vi "ReloaderMecanism.vi"() -> ()   [LabVIEW 2016]
uses:
  Globals/DIO.ctl
  Globals/Globals.vi
  Globals/InputValues.vi
panel:
  in  "wait":dbl
  out "Boolean":bool
  in  "Numeric":dbl
  out "Step even":bool
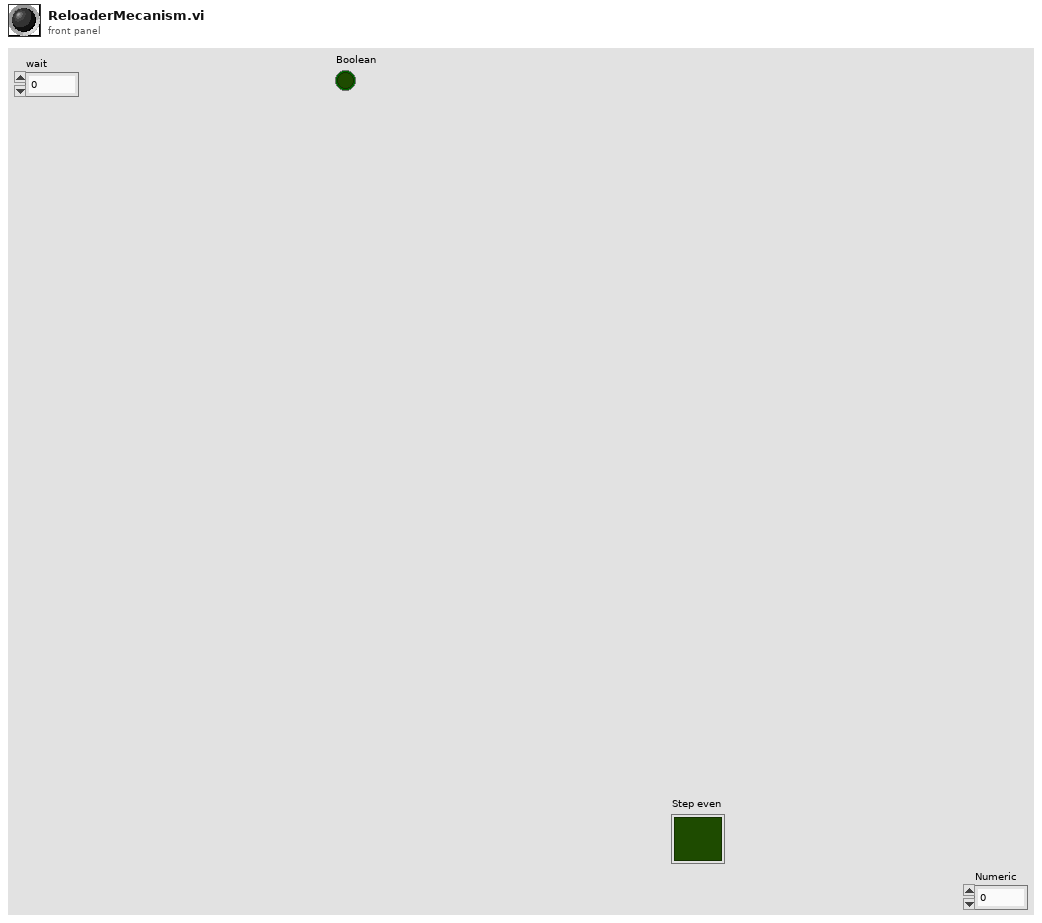
[diagram p1: front panel]
types:
  T1 = typedef "DIO.ctl" = string
  T2 = typedef "WPI_ServoDeviceRef.ctl" = cluster{"DeviceStatus":errorcluster, "PWM Channel":T3, "DeadBand":T4}
  T3 = typedef "FPGA_DIOPWMChannel.ctl" = enum8{"PWM 0", "PWM 1", "PWM 2", "PWM 3", "PWM 4", "PWM 5", "PWM 6", "PWM 7", "PWM 8", "PWM 9", "PWM MXP 0", "PWM MXP 1", "PWM MXP 2", "PWM MXP 3", "PWM MXP 4", "PWM MXP 5", "PWM MXP 6", "PWM MXP 7", "PWM MXP 8", "PWM MXP 9", "Invalid"}
  T4 = typedef "WPI_PWMDeadband.ctl" = cluster{"Name":string, "maxPositivePwm":i32, "minPositivePwm":i32, "centerPwm":i32, "maxNegativePwm":i32, "minNegativePwm":i32, "angularRange":u16}
  T5 = typedef "WPI_DigitalOutputDevRef.ctl" = cluster{"DIO Channel":T6, "DevStatus":errorcluster}
  T6 = typedef "FPGA_DIOChannel.ctl" = enum8{"DIO 0", "DIO 1", "DIO 2", "DIO 3", "DIO 4", "DIO 5", "DIO 6", "DIO 7", "DIO 8", "DIO 9", "DIO MXP 0", "DIO MXP 1", "DIO MXP 2", "DIO MXP 3", "DIO MXP 4", "DIO MXP 5", "DIO MXP 6", "DIO MXP 7", "DIO MXP 8", "DIO MXP 9", "DIO MXP 10", "DIO MXP 11", "DIO MXP 12", "DIO MXP 13", "DIO MXP 14", "DIO MXP 15", "SPI Port CS1", "SPI Port CS2", "SPI Port CS3", "SPI Port MISO", "SPI Port MOSI", "Invalid"}
  T7 = typedef "WPI_MotorControlDeviceRef.ctl" = cluster{"DeviceStatus":errorcluster, "Type":T8, "PWM":cluster{"PWM Channel":T3, "DeadBand":T4}, "CAN":cluster{"Device Number":u8, "SetOutput VI Ref":variant, "GetOutput VI Ref":variant, "Enable VI Ref":variant, "Disable VI Ref":variant, "Data":variant}, "Invert":bool}
  T8 = typedef "WPI_MotorControlType.ctl" = enum16{"PWM", "CAN"}
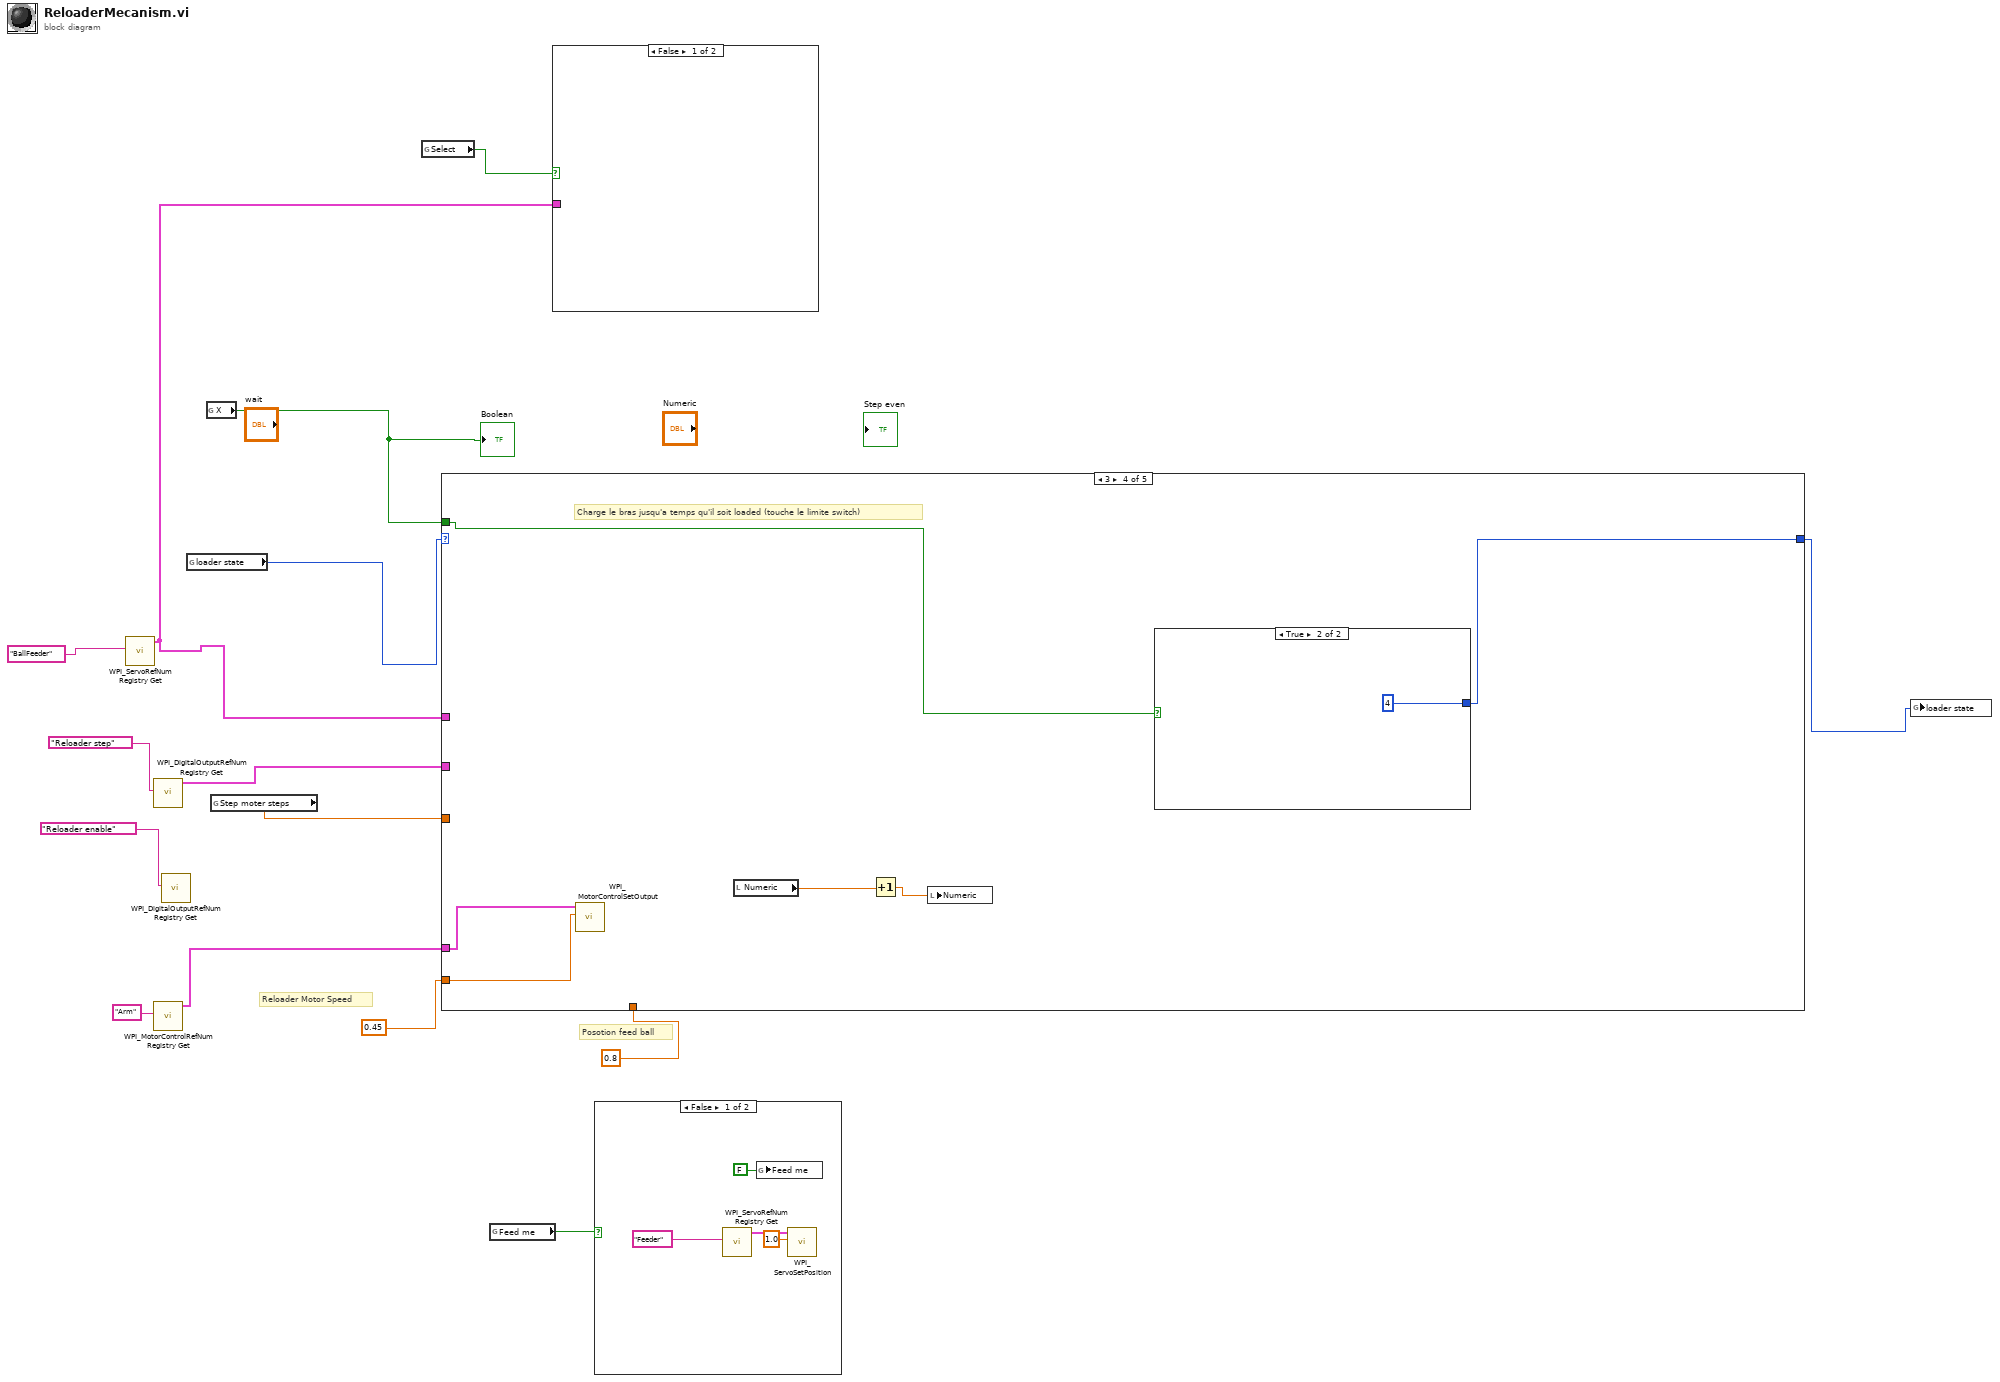
[diagram p0: block diagram]
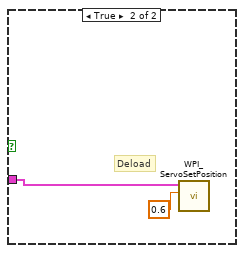
[diagram p2: hidden frame]
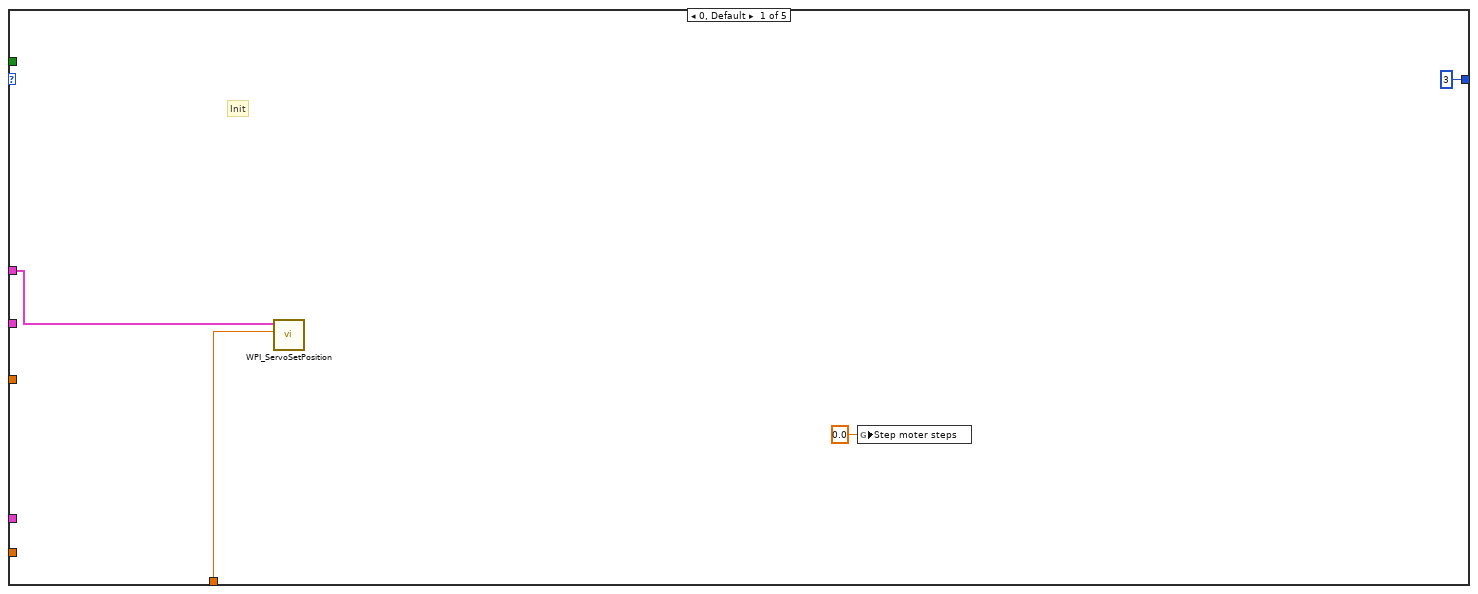
[diagram p4: hidden frame]
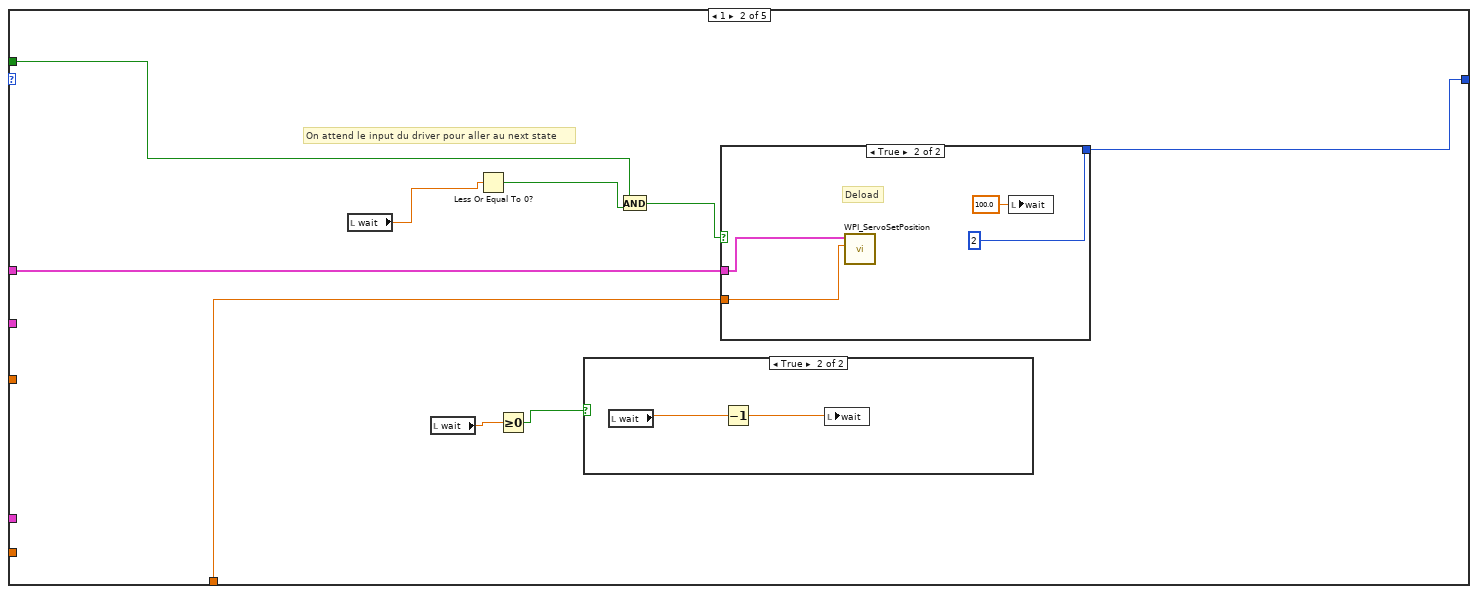
[diagram p5: hidden frame]
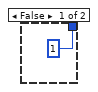
[diagram p7: hidden frame]
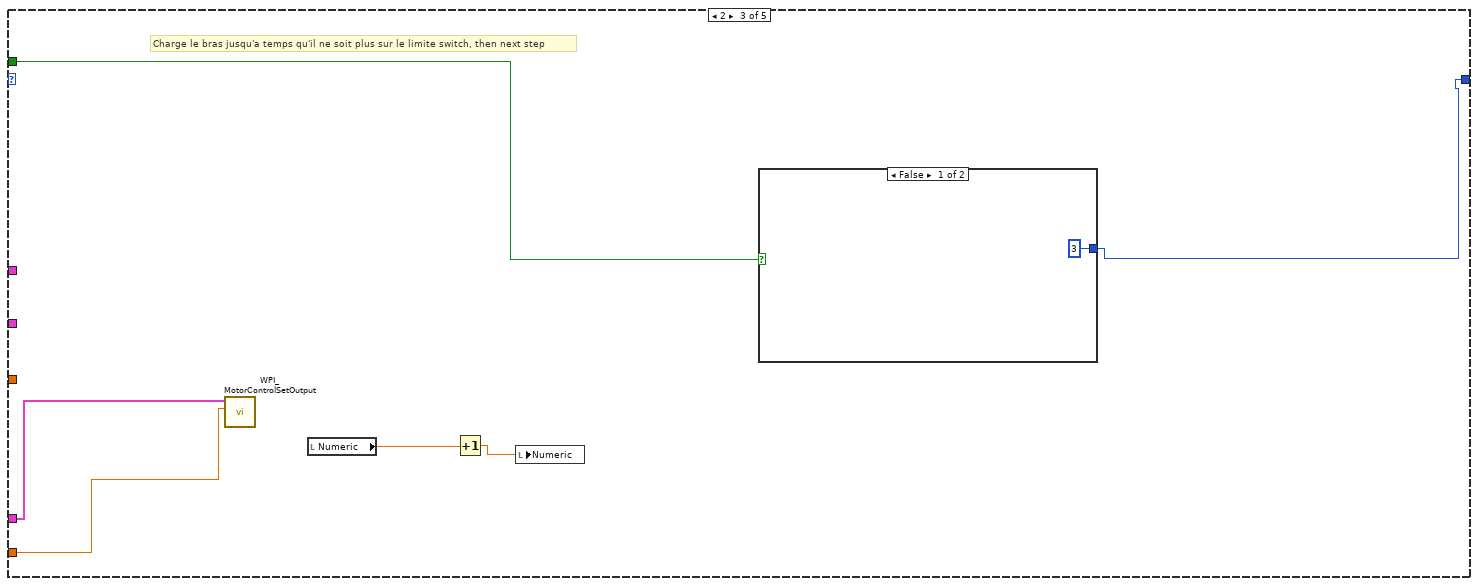
[diagram p8: hidden frame]
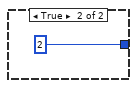
[diagram p9: hidden frame]
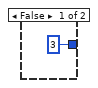
[diagram p10: hidden frame]
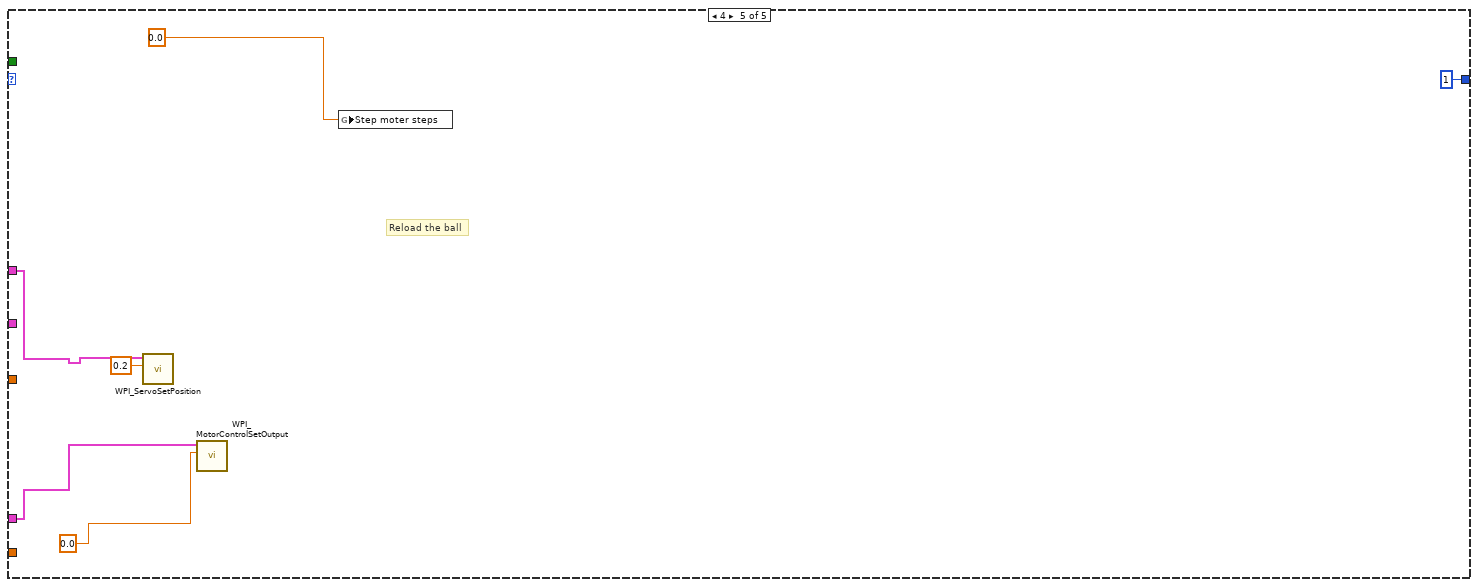
[diagram p11: hidden frame]
diagram:
  # "Posotion feed ball"
  # "Reloader Motor Speed"
  n1 = call <vilib>:"WPI_ServoRefNum Registry Get.vi"("refnum name"="BallFeeder") -> ("ServoDeviceRef"=w9:T2)  [unwired: 9 in, 1 out]
  n2 = call <vilib>:"WPI_DigitalOutputRefNum Registry Get.vi"("refnum name"=T1 "Reloader step" ("Combo Box")) -> ("DigitalOutputDevRef"=w13:T5)  [unwired: 9 in, 1 out]
  n3 = call <vilib>:"WPI_MotorControlRefNum Registry Get.vi"("refnum name"="Arm") -> ("MotorControlDevRef"=w6:T7)  [unwired: 9 in, 1 out]
  n4 = call <vilib>:"WPI_DigitalOutputRefNum Registry Get.vi"("refnum name"=T1 "Reloader enable" ("Combo Box")) -> ()  [unwired: 9 in, 2 out]
  n5 = global read "Globals.vi" "loader state"() -> (w2:i32)
  n6 = global read "InputValues.vi" "X"() -> (w3:bool)
  "Boolean" <- w3
  n7 = global read "Globals.vi" "Step moter steps"() -> (w8:dbl)
  n8 = global read "InputValues.vi" "Select"() -> (w10:bool)
  n9 = case shown="3" w2 {
    tunnel: [3 w28 w38 w47 1] -> w1
    tunnel: w3 -> [_ w24 w39 w46 _]
    tunnel: w8 -> [_ _ _ _ _]
    tunnel: w13 -> [_ _ _ _ _]
    tunnel: w9 -> [w17 w27 _ _ w54]
    tunnel: w6 -> [_ _ w37 w45 w53]
    tunnel: 0.45 ("Output") -> [_ _ w36 w44 _]
    tunnel: 0.8 ("Position") -> [w16 w26 _ _ _]
    frame 0, Default {
      # "Init"
      n10 = call <vilib>:"WPI_ServoSetPosition.vi"("Position"=w16, "ServoDeviceRef"=w17) -> ()  [unwired: 8 in, 2 out]
      n11 = global write "Globals.vi" "Step moter steps"(0.0 ("Step moter steps")) -> ()
    }
    frame 1 {
      # "On attend le input du driver pour aller au next state"
      n12 = local read "wait"() -> (w20:dbl)
      n13 = local read "wait"() -> (w22:dbl)
      n14 = Less Or Equal To 0?(x=w20) -> (x <= 0?=w25:bool)
      n15 = Greater Or Equal To 0?(x=w22) -> (x >= 0?=w21:bool)
      n16 = case shown="True" w21 {
        frame False {
        }
        frame True {
          n17 = local read "wait"() -> (w30:dbl)
          n18 = Decrement(x=w30) -> (x-1=w29:dbl)
          n19 = local write "wait"(w29) -> ()
        }
      }
      n20 = And(x=w24, y=w25) -> (x .and. y?=w23:bool)
      n21 = case shown="True" w23 {
        tunnel: [1 2] -> w28
        tunnel: w27 -> [_ w34]
        tunnel: w26 -> [_ w33]
        frame False {
        }
        frame True {
          # "Deload"
          n22 = call <vilib>:"WPI_ServoSetPosition.vi"("Position"=w33, "ServoDeviceRef"=w34) -> ()  [unwired: 8 in, 2 out]
          n23 = local write "wait"(100.0 ("wait")) -> ()
        }
      }
    }
    frame 2 {
      # "Charge le bras jusqu'a temps qu'il ne soit plus sur le limite switch, then next step"
      n24 = call <vilib>:"WPI_MotorControlSetOutput.vi"("Output"=w36, "MotorControlDevRef"=w37) -> ()  [unwired: 7 in, 3 out]
      n25 = local read "Numeric"() -> (w40:dbl)
      n26 = Increment(x=w40) -> (x+1=w41:dbl)
      n27 = local write "Numeric"(w41) -> ()
      n28 = case shown="False" w39 {
        tunnel: [3 2] -> w38
        frame False {
        }
        frame True {
        }
      }
    }
    frame 3 {
      # "Charge le bras jusqu'a temps qu'il soit loaded (touche le limite switch)"
      n29 = call <vilib>:"WPI_MotorControlSetOutput.vi"("Output"=w44, "MotorControlDevRef"=w45) -> ()  [unwired: 7 in, 3 out]
      n30 = local read "Numeric"() -> (w48:dbl)
      n31 = Increment(x=w48) -> (x+1=w49:dbl)
      n32 = local write "Numeric"(w49) -> ()
      n33 = case shown="True" w46 {
        tunnel: [3 4] -> w47
        frame False {
        }
        frame True {
        }
      }
    }
    frame 4 {
      # "Reload the ball"
      n34 = call <vilib>:"WPI_ServoSetPosition.vi"("Position"=0.2, "ServoDeviceRef"=w54) -> ()  [unwired: 8 in, 2 out]
      n35 = call <vilib>:"WPI_MotorControlSetOutput.vi"("Output"=0.0, "MotorControlDevRef"=w53) -> ()  [unwired: 7 in, 3 out]
      n36 = global write "Globals.vi" "Step moter steps"(0.0 ("Step moter steps")) -> ()
    }
  }
  n37 = global read "Globals.vi" "Feed me"() -> (w12:bool)
  n38 = case shown="False" w10 {
    tunnel: w9 -> [_ w58]
    frame False {
    }
    frame True {
      # "Deload"
      n39 = call <vilib>:"WPI_ServoSetPosition.vi"("Position"=0.6, "ServoDeviceRef"=w58) -> ()  [unwired: 8 in, 2 out]
    }
  }
  n40 = case shown="False" w12 {
    frame False {
      n41 = call <vilib>:"WPI_ServoRefNum Registry Get.vi"("refnum name"="Feeder") -> ("ServoDeviceRef"=w62:T2)  [unwired: 9 in, 1 out]
      n42 = global write "Globals.vi" "Feed me"(FALSE ("Feed me")) -> ()
      n43 = call <vilib>:"WPI_ServoSetPosition.vi"("Position"=1.0, "ServoDeviceRef"=w62) -> ()  [unwired: 8 in, 2 out]
    }
    frame True {
    }
  }
  n44 = global write "Globals.vi" "loader state"(w1) -> ()
